vi "LabVIEW_VI.vi"() -> ()   [LabVIEW 2019]
uses:
  89483c23-6296-43d6-9ccc-3825633ac357.vi
  <vilib>/numeric/Random Number (Range) DBL.vi
  8ed5f85a-e279-41a8-98b8-41f2e80916c9.vi
  155b3089-5dd6-4973-a0fd-1ad6976bf018.vi
  d7ff72c2-7c4d-40de-ab9a-9eb91e9960cf.vi
  a569d1ba-bd82-43fd-8394-a78add5a8c2f.vi
  4a742eb0-aa43-457c-b58c-e60e6cba93f9.vi
  f6be9f34-94d3-47c4-a592-19668ff3f23e.vi
  88238e0d-9124-481a-a212-2303bd455f48.vi
  72bce6ff-3756-4d9d-81ea-ac309b0d5ace.vi
  72a31ee0-8d40-4798-8ae2-afc8f18746f2.vi
  1f386d95-3959-433f-a59c-f0725bcc8a43.vi
panel:
  in  "ABORT CURRENT BATCH PROCESSING":bool
  out "Time remaining in process (seconds) 5":u8(slide) scale=0.0..255.0
  out "On 7":bool
  out "Completed batch - ready for packing":string[](array[string])
  out "Roasting Temperature":dbl(slide) scale=100.0..300.0
  out "Time remaining in process (seconds) 4":u8(slide) scale=0.0..255.0
  out "Current batch after sorting":string[](array[string])
  out "On 6":bool
  out "On 5":bool
  out "Time remaining in process (seconds) 3":u8(slide) scale=0.0..255.0
  out "Current batch after hulling":string[](array[string])
  out "On 4":bool
  out "Time remaining in process (seconds) 2":u8(slide) scale=0.0..255.0
  out "Current batch after cleaning":string[](array[string])
  out "On 3":bool
  out "Time remaining in process (seconds)":u8(slide) scale=0.0..255.0
  out "Current batch after recombination":string[](array[string])
  out "Estimated internal temperature of batch":dbl(slide) scale=0.0..100.0
  out "Sub-Batch - 2 (After washing)":string[](array[string])
  out "On 2":bool
  out "Washing Tank":dbl(slide) scale=0.0..10.0
  out "Sub-Batch - 2 (After fermentaion)":string[](array[string])
  out "Estimated Moisture content of batch(%)":dbl(knob) scale=0.0..100.0
  out "On 1":bool
  out "Sub-Batch - 2 (After pulping)":string[](array[string])
  out "Sub-Batch - 2":string[](array[string])
  out "On":bool
  out "Sub-Batch - 1":string[](array[string])
  out "Receiving Tank":dbl(slide) scale=0.0..1000.0
  out "Current Batch being processed":string[](array[string])
  out "Price of Coffee\n(Per Kilogram)":string
  out "Price of Coffee Decimel":dbl
  # "Batch ID"
  # "Total\nWeight (Kg)"
  # "Expected Cost ($)"
  # "Type of Coffee Cherries"
  # "Entire batch is added to the Receiving Tank"
  # "1. RECEIVING"
  # "Processing"
  # "Anything that sinks is sent to the \npulping process and the tank is emptied"
  # "Anything that floats is sent \ndirectly to the drying proccess (Around 1-10% of total weight)"
  # "Batch ID"
  # "Total Weight \n(Dried Cherries/Impurities)(Kg)"
  # "Expected Cost ($)"
  # "Type of Coffee Cherries"
  # "Batch ID"
  # "Total Weight \n(Ripe Cherries))(Kg)"
  # "Expected Cost ($)"
  # "Type of Coffee Cherries"
  # "The 1st sub-batch is sent directly to the drying process"
  # "The 2nd sub-batch containing the Ripe \ncherries are then sent to the pulping process"
  # "The sub-batch is fermented to weaken the mucilage surronding beans"
  # "2. PULPING"
  # "Processing"
  # "3. FERMENTATION"
  # "Batch ID"
  # "Total Weight (Pulp removed) (Kg)"
  # "Expected Cost ($)"
  # "Type of Coffee Cherries"
  # "The pulping process removes most of the cherry leaving the bean\n\nDepending on the cherry type, a different amount of beans are yielded after this process"
  # "Arabica Coffee (15-19%)\nRobusta (18-23%)\nExcelsa (25 - 30%)\nLibericia (26-31%)"
  # "Batch ID"
  # "Total Weight (Fermented) (Kg)"
  # "Expected Cost ($)"
  # "Type of Coffee Cherries"
  # "Moisture Content (%)"
  # "The sub-batches are then recombined into the same batch again, and are dried together, resulting in dry husk coffee (from sub-batch 1) and dry parchment coffee (from sub-batch 2)"
  # "4. WASHING"
  # "Processing"
  # "5. DRYING"
  # "Processing"
  # "The batch is dried in an industrial dehumidifer in a factory, and the temperature is kept around 37 - 45 C to prevent case hardening of the beans. They are dried until their moisture content has reached 10-12%"
  # "Time remaining in process (seconds)"
  # "Batch ID"
  # "Total Weight (Washed) (Kg)"
  # "Expected Cost ($)"
  # "Type of Coffee Cherries"
  # "Moisture Content (%)"
  # "Batch ID"
  # "Total Weight (KG)"
  # "Expected Cost ($)"
  # "Type of Coffee Cherries"
  # "Moisture Content (%)"
  # "The sub-batch is then washed to removed the weakened mucilage, \nresulting in wet parchment coffee"
  # "6. CLEANING"
  # "Processing"
  # "7. HULLING"
  # "Processing"
  # "The batch may still contain some rocks, pebbles, twigs, etc. So one last final cleaning process is ran on the batch via the use of hoppers, screen and magnetic seperators"
  # "Finally, the batch is now hulled, to remove the husks and dry parchments attached, resulting in now pure coffee beans remaining"
  # "Time remaining in process (seconds)"
  # "Time remaining in process (seconds)"
  # "Batch ID"
  # "Total Weight (KG)"
  # "Expected Cost ($)"
  # "Type of Coffee Cherries"
  # "Moisture Content (%)"
  # "Batch ID"
  # "Total Weight (KG)"
  # "Expected Cost ($)"
  # "Type of Coffee Cherries"
  # "Moisture Content (%)"
  # "9. ROASTING"
  # "Processing"
  # "8. SORTING"
  # "Processing"
  # "The coffee beans are now sorted to remove any defective, insect-attacked or miscoloured beans via the use of electronic and manual sorting within the factory, leaving only desirable coffee beans in the batch"
  # "Time remaining in process (seconds)"
  # "Time remaining in process (seconds)"
  # "Batch ID"
  # "Total Weight (KG)"
  # "Actual Cost ($)"
  # "Expected Cost ($)"
  # "Moisture Content (%)"
  # "Batch ID"
  # "Total Weight (KG)"
  # "Expected Cost ($)"
  # "Type of Coffee Cherries"
  # "Moisture Content (%)"
  # "Finally, since only pure coffee beans remain in the batch, they are roasted at a temperature around 200 - 250C, losing around 1-2% of moisture in the process, and subsequently around 1-2% weight loss"
  # "Since majority of the batch was wet-processed, there will be little undesirable beans remaining in the batch"
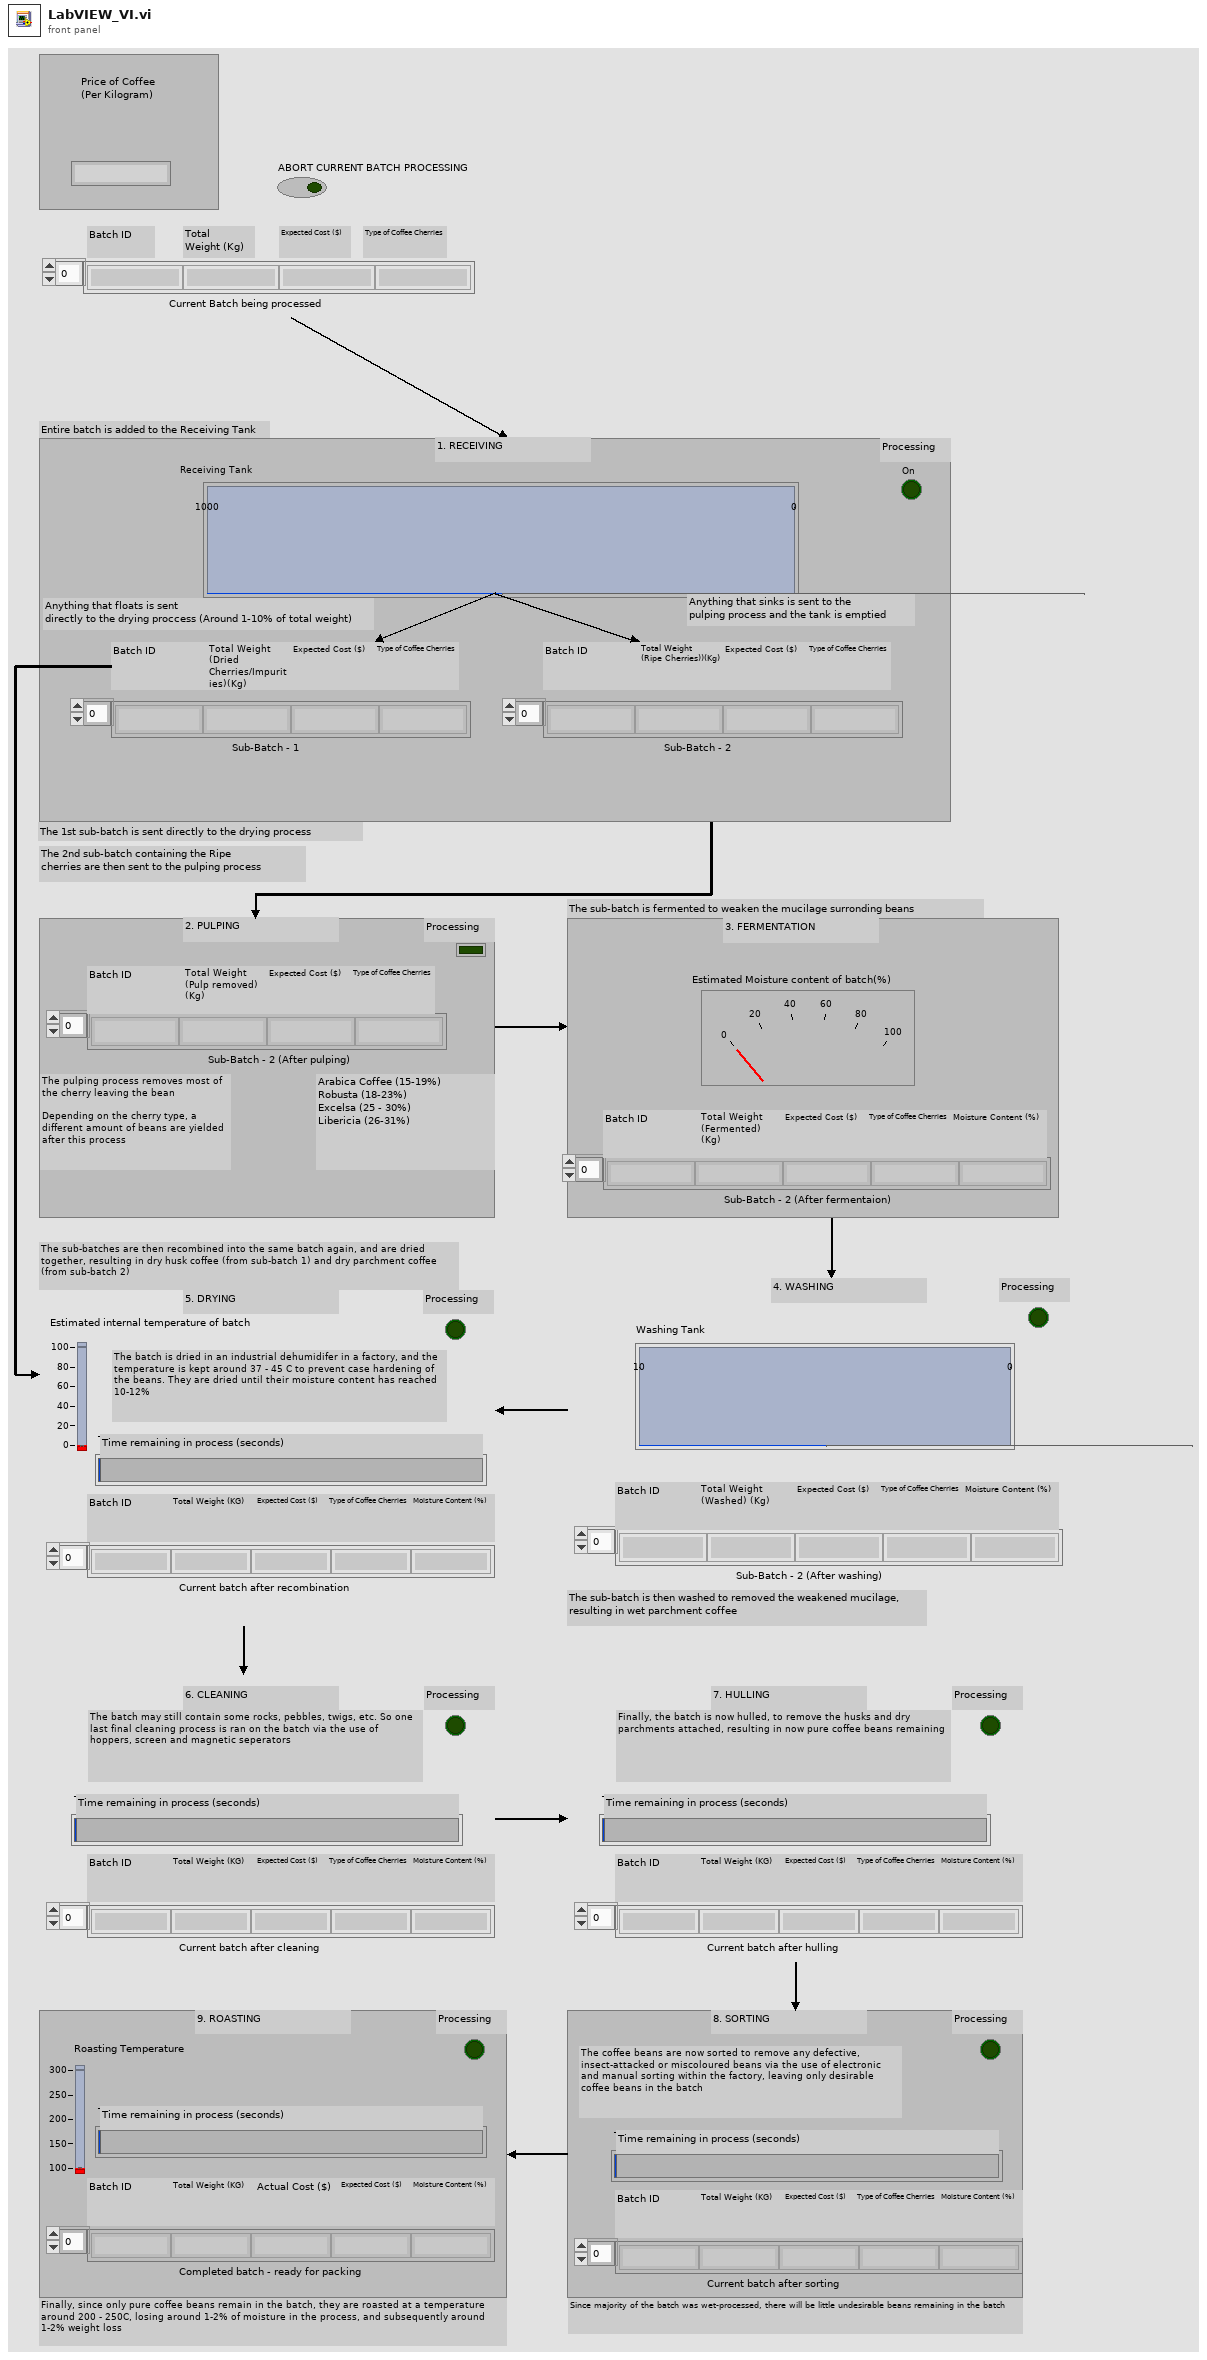
[diagram p1: front panel]
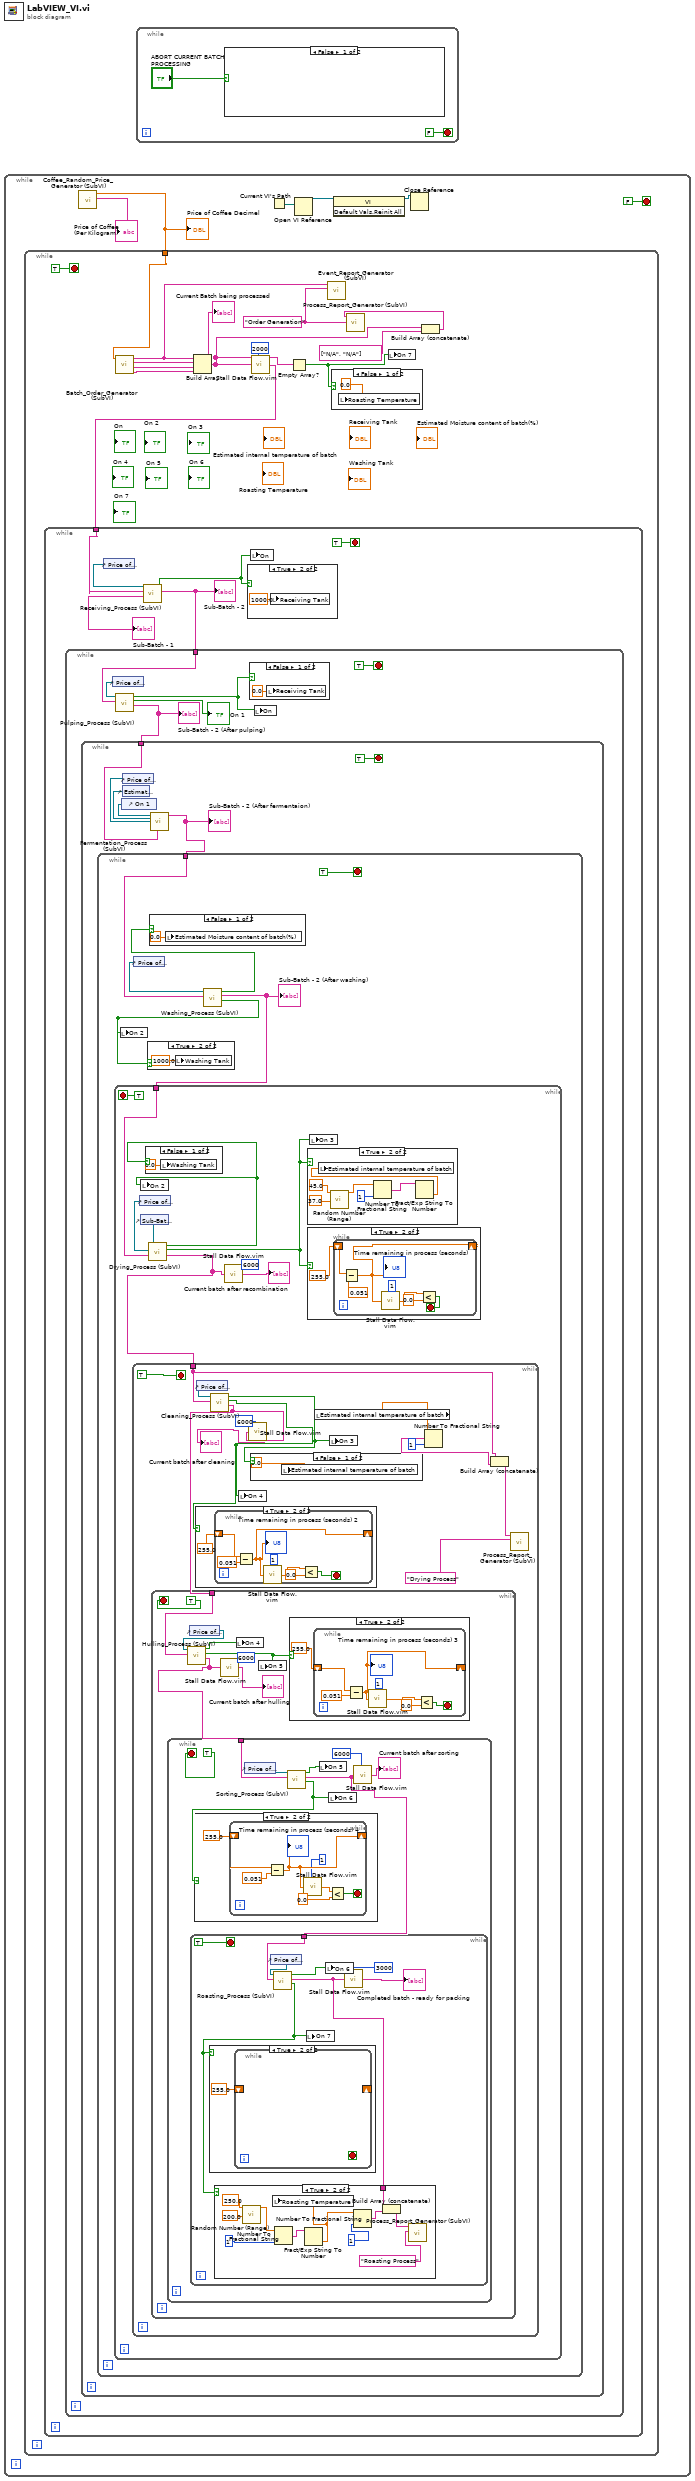
[diagram p0: block diagram]
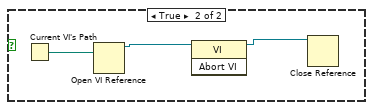
[diagram p2: hidden frame]
diagram:
  n1 = while {
    stop <- FALSE stop-if-true
    n2 = call "Coffee_Random_Price_Generator (SubVI).vi"() -> ("String"=→"Price of Coffee\n(Per Kilogram)":string, "number"=w6:dbl)  [unwired: 10 in]
    "Price of Coffee Decimel" <- w6
    n3 = while {
      tunnel: w6 -> [w14]
      stop <- TRUE stop-if-true
      w11 = "Order Generation" ("element")
      n4 = call "Batch_Order_Generator (SubVI).vi"("Price of Coffee Decimel"=w14) -> ("String 2"=w18:string, "String 3"=w19:string, "String 4"=w12:string, "String"=w13:string)  [unwired: 7 in]
      n5 = Build Array(w12, w19, w18, w13) -> (w9:string[])
      "Current Batch being processed" <- w9
      n6 = call "Stall Data Flow.vim"("value in"=w9, "milliseconds to wait"=u32 2000) -> ("value out"=w16:string[])  [unwired: 1 out]
      n7 = while {
        tunnel: w16 -> [w23]
        stop <- TRUE stop-if-true
        n8 = control-ref of="Price of Coffee Decimel"() -> (w24:refnum<vi>)
        n9 = call "Receiving_Process (SubVI).vi"("value in"=w23, "Digital in"=w24) -> ("Array"=→"Sub-Batch - 1":string[], "Array 2"=w22:string[], "Boolean"=w26:bool)  [unwired: 7 in]
        "Sub-Batch - 2" <- w22
        n10 = while {
          tunnel: w22 -> [w29]
          stop <- TRUE stop-if-true
          n11 = control-ref of="Price of Coffee Decimel"() -> (w30:refnum<vi>)
          n12 = call "Pulping_Process (SubVI).vi"("Array in"=w29, "Digital in"=w30) -> ("Array out"=w28:string[], "Boolean"=→"On 1":bool, "empty?"=w31:bool)  [unwired: 7 in]
          "Sub-Batch - 2 (After pulping)" <- w28
          n13 = while {
            tunnel: w28 -> [w35]
            stop <- TRUE stop-if-true
            n14 = control-ref of="On 1"() -> (w37:refnum<vi>)
            n15 = control-ref of="Price of Coffee Decimel"() -> (w36:refnum<vi>)
            n16 = control-ref of="Estimated Moisture content of batch(%)"() -> (w38:refnum<vi>)
            n17 = call "Fermentation_Process (SubVI).vi"("Array in"=w35, "Temperature Guage"=w38, "reference in"=w36, "Boolean in"=w37) -> ("Array out"=w34:string[])  [unwired: 7 in]
            "Sub-Batch - 2 (After fermentaion)" <- w34
            n18 = while {
              tunnel: w34 -> [w44]
              stop <- TRUE stop-if-true
              n19 = control-ref of="Price of Coffee Decimel"() -> (w42:refnum<vi>)
              n20 = call "Washing_Process (SubVI).vi"("Array in"=w44, "Digital in"=w42) -> ("Boolean"=w43:bool, "Array out"=w41:string[], "empty?"=w40:bool)  [unwired: 7 in]
              "Sub-Batch - 2 (After washing)" <- w41
              n21 = while {
                tunnel: w41 -> [w53]
                stop <- TRUE stop-if-true
                n22 = control-ref of="Price of Coffee Decimel"() -> (w49:refnum<vi>)
                n23 = control-ref of="Sub-Batch - 1"() -> (w50:refnum<vi>)
                n24 = call "Drying_Process (SubVI).vi"("Array 2"=w53, "reference in"=w49, "Array in"=w50) -> ("Array"=w46:string[], "Boolean"=w51:bool, "empty?"=w48:bool)  [unwired: 6 in]
                n25 = while {
                  tunnel: w46 -> [w58]
                  stop <- TRUE stop-if-true
                  n26 = control-ref of="Price of Coffee Decimel"() -> (w65:refnum<vi>)
                  n27 = call "Cleaning_Process (SubVI).vi"("Array in"=w58, "Digital in"=w65) -> ("Array out"=w55:string[], "Boolean"=w64:bool, "empty?"=w63:bool)  [unwired: 7 in]
                  n28 = while {
                    tunnel: w55 -> [w73]
                    stop <- TRUE stop-if-true
                    n29 = control-ref of="Price of Coffee Decimel"() -> (w70:refnum<vi>)
                    n30 = call "Hulling_Process (SubVI).vi"("Array in"=w73, "Digital in"=w70) -> ("Array out"=w68:string[], "Boolean"=w71:bool, "empty?"=w72:bool)  [unwired: 7 in]
                    n31 = while {
                      tunnel: w68 -> [w80]
                      stop <- TRUE stop-if-true
                      n32 = control-ref of="Price of Coffee Decimel"() -> (w81:refnum<vi>)
                      n33 = call "Sorting_Process (SubVI).vi"("Array in"=w80, "Digital in"=w81) -> ("Boolean"=w79:bool, "Array out"=w76:string[], "empty?"=w82:bool)  [unwired: 7 in]
                      n34 = while {
                        tunnel: w76 -> [w85]
                        stop <- TRUE stop-if-true
                        n35 = control-ref of="Price of Coffee Decimel"() -> (w89:refnum<vi>)
                        n36 = call "Roasting_Process (SubVI).vi"("Array in"=w85, "Digital in"=w89) -> ("Boolean"=w88:bool, "Array out"=w84:string[], "empty?"=w90:bool)  [unwired: 7 in]
                        n37 = case shown="True" w88 {
                          frame False {
                          }
                          frame True {
                            n38 = while {
                              shift-right: [w103] -> _
                              shift-left: 255.0 -> [w104]
                              stop <- w109 stop-if-true
                              n39 = Subtract(x=w104, y=0.051) -> (x-y=w103:dbl)
                              "Time remaining in process (seconds) 5" <- w103
                              n40 = call "Stall Data Flow.vim"("value in"=w103, "milliseconds to wait"=u32 1) -> ("value out"=w107:dbl)  [unwired: 1 out]
                              n41 = Less?(x=w107, y=0.0) -> (x < y?=w109:bool)
                            }
                          }
                        }
                        n42 = case shown="True" w88 {
                          tunnel: w84 -> [_ w93]
                          frame False {
                          }
                          frame True {
                            n43 = call-poly <vilib>:"Random Number (Range).vi"("lower bound (0)"=200.0, "upper bound (100)"=250.0) -> ("number"=w98:dbl)  [unwired: 9 in]
                            n44 = Number To Fractional String(number=w98, precision (6)=i16 1) -> (F-format string=w97:string)  [unwired: 2 in]
                            n45 = Fract/Exp String To Number(string=w97) -> (number=w96:dbl)  [unwired: 3 in, 1 out]
                            n46 = local write "Roasting Temperature"(w96) -> ()
                            n47 = Number To Fractional String(number=w96, precision (6)=i16 1) -> (F-format string=w94:string)  [unwired: 2 in]
                            n48 = Build Array (concatenate)(w93, w94) -> (w91:string[])
                            n49 = call "Process_Report_Generator (SubVI).vi"("Process Name"="Roasting Process", "Process Information"=w91) -> ()  [unwired: 10 in]
                          }
                        }
                        n50 = local write "On 7"(w88) -> ()
                        n51 = local write "On 6"(w90) -> ()
                        n52 = call "Stall Data Flow.vim"("value in"=w84, "milliseconds to wait"=u32 3000) -> ("value out"=→"Completed batch - ready for packing":string[])  [unwired: 1 out]
                      }
                      n53 = case shown="True" w79 {
                        frame False {
                        }
                        frame True {
                          n54 = while {
                            shift-right: [w113] -> _
                            shift-left: 255.0 -> [w111]
                            stop <- w117 stop-if-true
                            n55 = Subtract(x=w111, y=0.051) -> (x-y=w113:dbl)
                            "Time remaining in process (seconds) 4" <- w113
                            n56 = call "Stall Data Flow.vim"("value in"=w113, "milliseconds to wait"=u32 1) -> ("value out"=w115:dbl)  [unwired: 1 out]
                            n57 = Less?(x=w115, y=0.0) -> (x < y?=w117:bool)
                          }
                        }
                      }
                      n58 = local write "On 5"(w82) -> ()
                      n59 = local write "On 6"(w79) -> ()
                      n60 = call "Stall Data Flow.vim"("value in"=w76, "milliseconds to wait"=u32 6000) -> ("value out"=→"Current batch after sorting":string[])  [unwired: 1 out]
                    }
                    n61 = call "Stall Data Flow.vim"("value in"=w68, "milliseconds to wait"=u32 6000) -> ("value out"=→"Current batch after hulling":string[])  [unwired: 1 out]
                    n62 = local write "On 4"(w72) -> ()
                    n63 = local write "On 5"(w71) -> ()
                    n64 = case shown="True" w71 {
                      frame False {
                      }
                      frame True {
                        n65 = while {
                          shift-right: [w119] -> _
                          shift-left: 255.0 -> [w120]
                          stop <- w122 stop-if-true
                          n66 = Subtract(x=w120, y=0.051) -> (x-y=w119:dbl)
                          "Time remaining in process (seconds) 3" <- w119
                          n67 = call "Stall Data Flow.vim"("value in"=w119, "milliseconds to wait"=u32 1) -> ("value out"=w124:dbl)  [unwired: 1 out]
                          n68 = Less?(x=w124, y=0.0) -> (x < y?=w122:bool)
                        }
                      }
                    }
                  }
                  n69 = case shown="True" w64 {
                    frame False {
                    }
                    frame True {
                      n70 = while {
                        shift-right: [w128] -> _
                        shift-left: 255.0 -> [w132]
                        stop <- w129 stop-if-true
                        n71 = Subtract(x=w132, y=0.051) -> (x-y=w128:dbl)
                        "Time remaining in process (seconds) 2" <- w128
                        n72 = call "Stall Data Flow.vim"("value in"=w128, "milliseconds to wait"=u32 1) -> ("value out"=w130:dbl)  [unwired: 1 out]
                        n73 = Less?(x=w130, y=0.0) -> (x < y?=w129:bool)
                      }
                    }
                  }
                  n74 = local write "On 4"(w64) -> ()
                  n75 = call "Stall Data Flow.vim"("value in"=w55, "milliseconds to wait"=u32 6000) -> ("value out"=→"Current batch after cleaning":string[])  [unwired: 1 out]
                  n76 = case shown="False" w63 {
                    frame False {
                      n77 = local write "Estimated internal temperature of batch"(0.0 ("Estimated internal temperature of batch")) -> ()
                    }
                    frame True {
                    }
                  }
                  n78 = local read "Estimated internal temperature of batch"() -> (w59:dbl)
                  n79 = local write "On 3"(w63) -> ()
                  n80 = Number To Fractional String(number=w59, precision (6)=i16 1) -> (F-format string=w60:string)  [unwired: 2 in]
                  n81 = Build Array (concatenate)(w58, w60) -> (w57:string[])
                  n82 = call "Process_Report_Generator (SubVI).vi"("Process Name"="Drying Process", "Process Information"=w57) -> ()  [unwired: 10 in]
                }
                n83 = local write "On 2"(w48) -> ()
                n84 = case shown="False" w48 {
                  frame False {
                    n85 = local write "Washing Tank"(0.0 ("Washing Tank")) -> ()
                  }
                  frame True {
                  }
                }
                n86 = call "Stall Data Flow.vim"("value in"=w46, "milliseconds to wait"=u32 6000) -> ("value out"=→"Current batch after recombination":string[])  [unwired: 1 out]
                n87 = case shown="True" w51 {
                  frame False {
                  }
                  frame True {
                    n88 = call-poly <vilib>:"Random Number (Range).vi"("lower bound (0)"=37.0, "upper bound (100)"=45.0) -> ("number"=w146:dbl)  [unwired: 9 in]
                    n89 = Number To Fractional String(number=w146, precision (6)=i16 1) -> (F-format string=w145:string)  [unwired: 2 in]
                    n90 = Fract/Exp String To Number(string=w145) -> (number=w144:dbl)  [unwired: 3 in, 1 out]
                    n91 = local write "Estimated internal temperature of batch"(w144) -> ()
                  }
                }
                n92 = case shown="True" w51 {
                  frame False {
                  }
                  frame True {
                    n93 = while {
                      shift-right: [w136] -> _
                      shift-left: 255.0 ("x") -> [w139]
                      stop <- w141 stop-if-true
                      n94 = Subtract(x=w139, y=0.051) -> (x-y=w136:dbl)
                      "Time remaining in process (seconds)" <- w136
                      n95 = call "Stall Data Flow.vim"("value in"=w136, "milliseconds to wait"=u32 1) -> ("value out"=w138:dbl)  [unwired: 1 out]
                      n96 = Less?(x=w138, y=0.0) -> (x < y?=w141:bool)
                    }
                  }
                }
                n97 = local write "On 3"(w51) -> ()
              }
              n98 = local write "On 2"(w43) -> ()
              n99 = case shown="True" w43 {
                frame False {
                }
                frame True {
                  n100 = local write "Washing Tank"(1000.0 ("Washing Tank")) -> ()
                }
              }
              n101 = case shown="False" w40 {
                frame False {
                  n102 = local write "Estimated Moisture content of batch(%)"(0.0 ("Estimated Moisture content of batch(%)")) -> ()
                }
                frame True {
                }
              }
            }
          }
          n103 = case shown="False" w31 {
            frame False {
              n104 = local write "Receiving Tank"(0.0 ("Receiving Tank")) -> ()
            }
            frame True {
            }
          }
          n105 = local write "On"(w31) -> ()
        }
        n106 = case shown="True" w26 {
          frame False {
          }
          frame True {
            n107 = local write "Receiving Tank"(1000.0 ("Receiving Tank")) -> ()
          }
        }
        n108 = local write "On"(w26) -> ()
      }
      n109 = Empty Array?(array=w9) -> (empty?=w15:bool)
      n110 = call "Event_Report_Generator (SubVI).vi"("Process Name"=w11, "Booking ID"=w12) -> ()  [unwired: 10 in]
      n111 = case shown="False" w15 {
        frame False {
          n112 = local write "Roasting Temperature"(0.0 ("Roasting Temperature")) -> ()
        }
        frame True {
        }
      }
      n113 = local write "On 7"(w15) -> ()
      n114 = Build Array (concatenate)(w9, string[] ["N/A", "N/A"] ("array")) -> (w8:string[])
      n115 = call "Process_Report_Generator (SubVI).vi"("Process Name"=w11, "Process Information"=w8) -> ()  [unwired: 10 in]
    }
    n116 = Current VI's Path() -> (path=w3:path)
    n117 = Open VI Reference(vi path=w3) -> (vi reference=w1:refnum<vi>)  [unwired: 5 in, 1 out]
    n118 = invoke class="VI" method="Default Vals.Reinit All"(reference=w1) -> (reference out=w2:refnum<vi>)  [unwired: 2 in, 2 out]
    n119 = Close Reference(reference=w2) -> ()  [unwired: 1 in, 1 out]
  }
  n120 = while {
    stop <- FALSE stop-if-true
    n121 = case shown="False" "ABORT CURRENT BATCH PROCESSING" {
      frame False {
      }
      frame True {
        n122 = Current VI's Path() -> (path=w156:path)
        n123 = Open VI Reference(vi path=w156) -> (vi reference=w158:refnum<vi>)  [unwired: 5 in, 1 out]
        n124 = invoke class="VI" method="Abort VI"(reference=w158) -> (reference out=w157:refnum<vi>)  [unwired: 2 in, 2 out]
        n125 = Close Reference(reference=w157) -> ()  [unwired: 1 in, 1 out]
      }
    }
  }
